vi "PH_Interaction.set PCS System.vi"() -> (0 "Enum":T1(ring))   [LabVIEW 2014, in "PH_Common.lvlib"]
doc: "This VI sets the PCS System. Default is \"PCS\"."
uses:
  PH_Common.lvlib
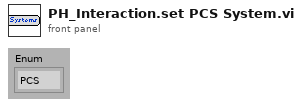
[diagram p1: front panel]
types:
  T1 = enum16{"PCS", "Laser", "Vision", "PP", "Special", "Beckhoff"}
  T2 = enum16{"PCS", "Laser", "Vision", "PP", "Special"}
  T3 = enum16{"PCS", "Laser", "PP", "Special", "Beckhoff"}
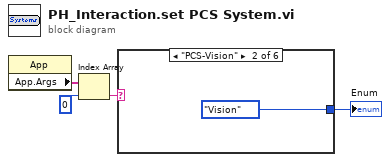
[diagram p0: block diagram]
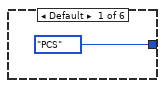
[diagram p2: hidden frame]
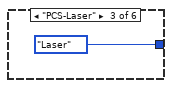
[diagram p3: hidden frame]
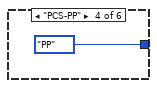
[diagram p4: hidden frame]
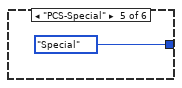
[diagram p5: hidden frame]
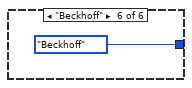
[diagram p6: hidden frame]
diagram:
  n1 = property class="App"() -> ("App.Args"=w4:string[])  [unwired: 2 in, 2 out]
  n2 = Index Array(array=w4, index=0) -> (element=w2:string)
  n3 = case shown="\"PCS-Vision\"" w2 {
    tunnel: [T2."PCS" ("Enum") T2."Vision" ("Enum") T2."Laser" ("Enum") T2."PP" ("Enum") T1."Special" ("Enum") T3."Beckhoff" ("Enum")] -> w1
    frame Default {
    }
    frame "PCS-Vision" {
    }
    frame "PCS-Laser" {
    }
    frame "PCS-PP" {
    }
    frame "PCS-Special" {
    }
    frame "Beckhoff" {
    }
  }
  "Enum" <- w1
